vi "Log_Test.vi"() -> ()   [LabVIEW 2021]
panel:
  out "x-y":dbl
  out "Array":T1(array[cluster])
  out "string array":string[](array[string])
  out "XY Graph":T2(graph)
  in  "Stop":bool
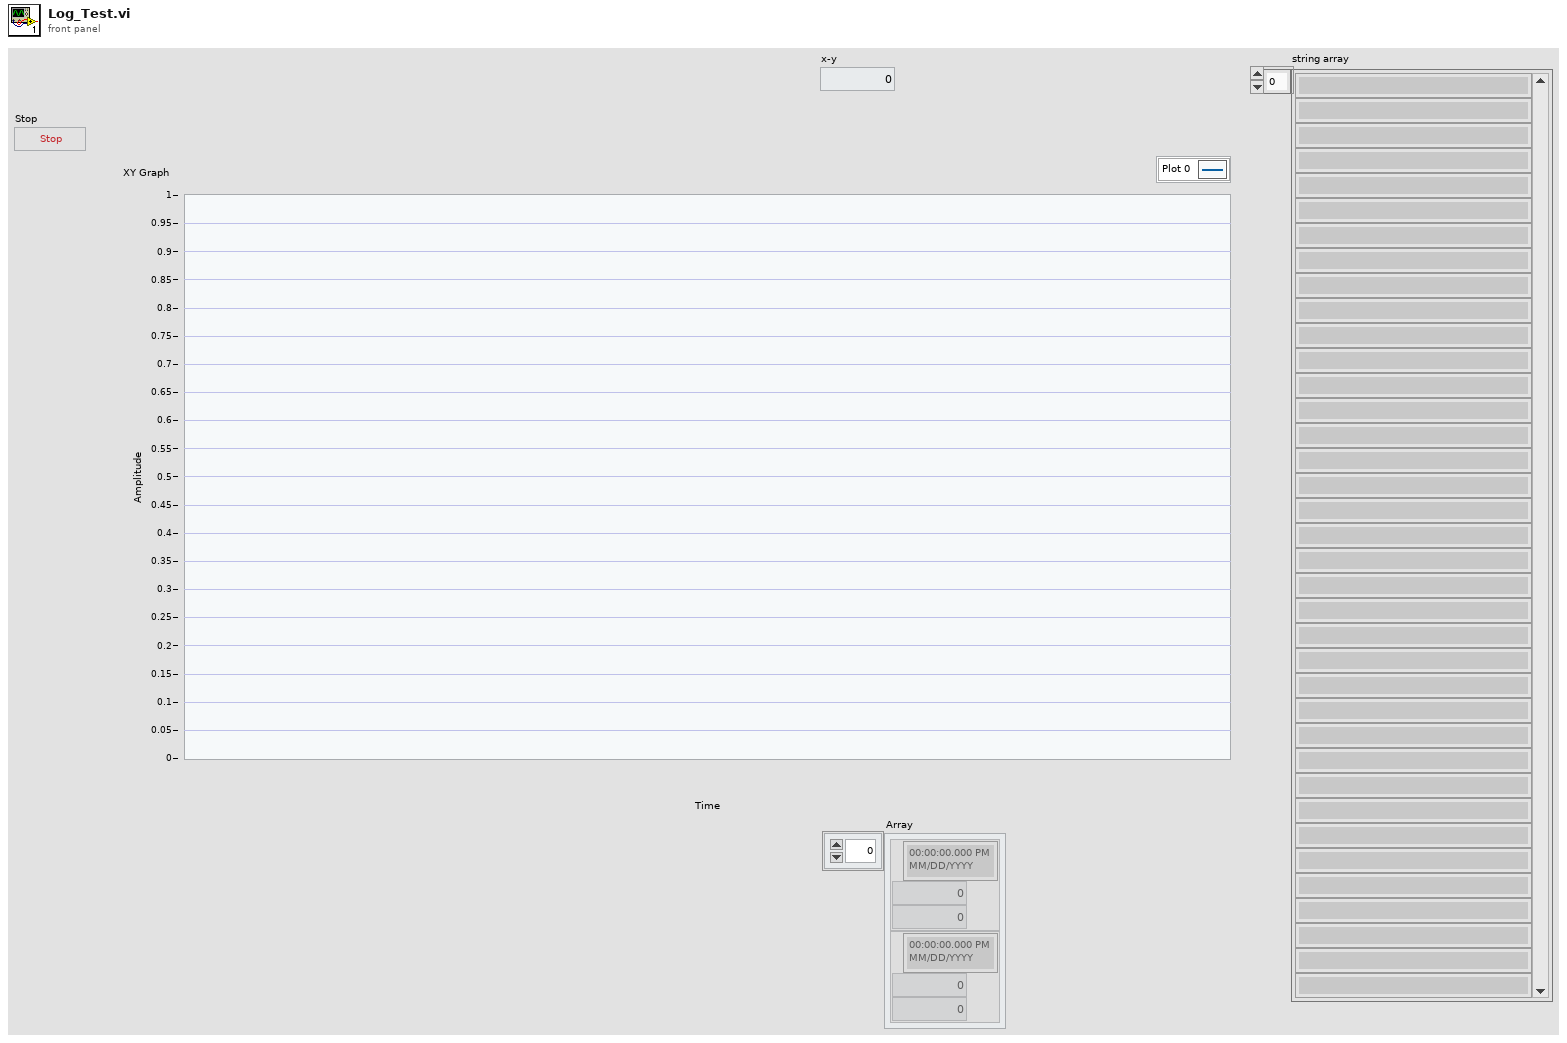
[diagram p1: front panel]
types:
  T1 = cluster{timestamp, "Numeric":dbl, "Numeric":dbl}[]
  T2 = cluster{"seconds since 1Jan1904":timestamp, "number: 0 to 1":dbl, "number: 0 to 1":dbl}[]
  T3 = enum16{"open", "replace", "create", "open or create", "replace or create", "replace or create with confirmation"}
  T4 = cluster{"seconds since 1Jan1904":timestamp, "number: 0 to 1":dbl, "number: 0 to 1":dbl}
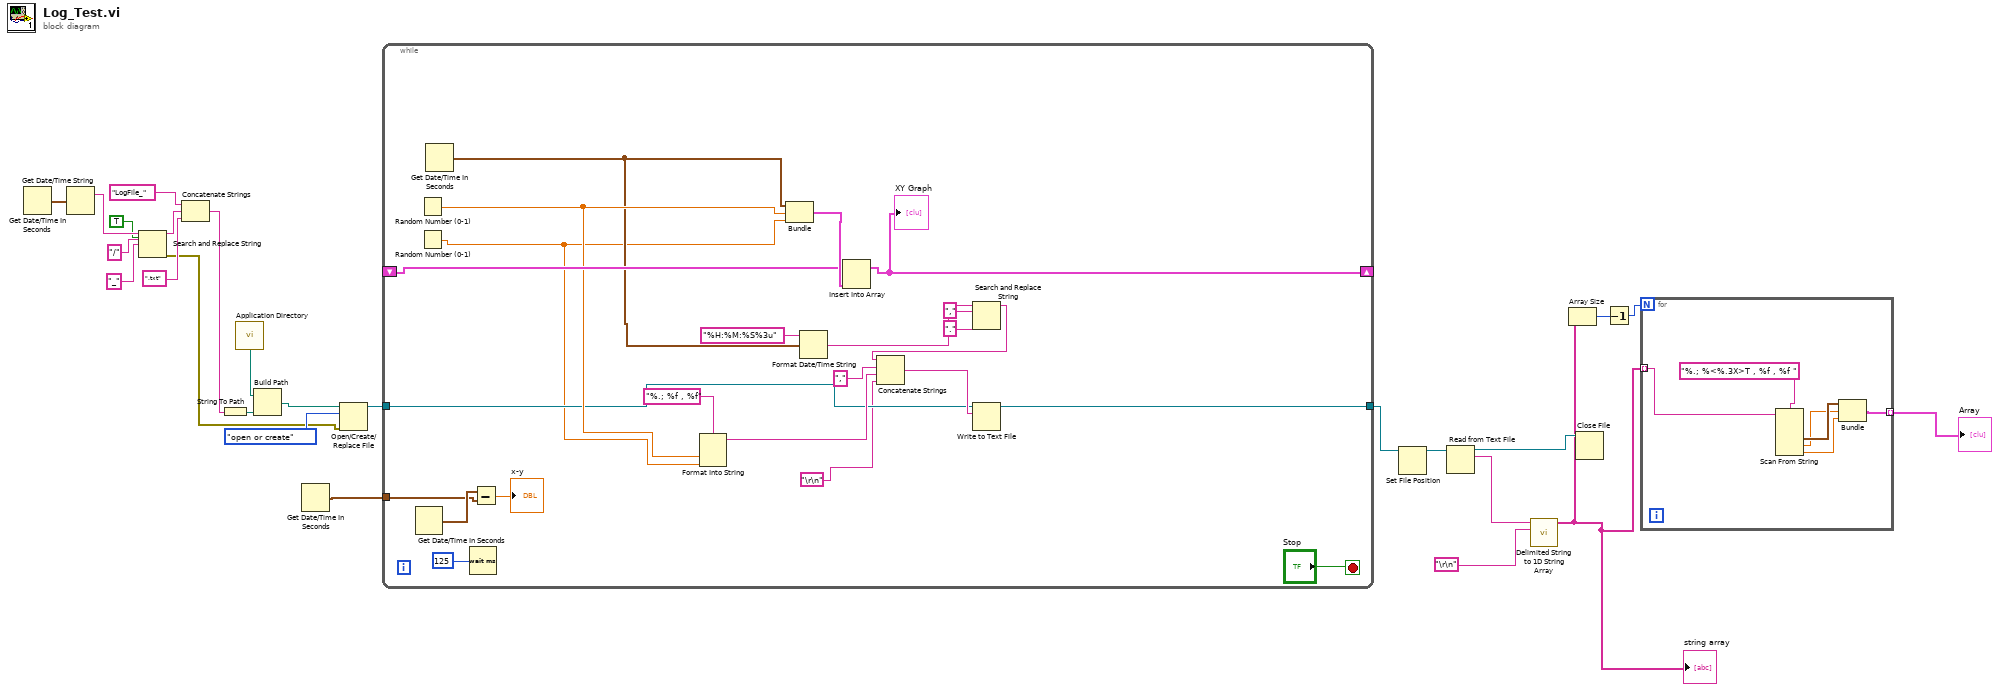
[diagram p0: block diagram]
diagram:
  n1 = Get Date/Time In Seconds() -> (seconds since 1Jan1904=w20:timestamp)
  n2 = Get Date/Time String(seconds (now)=w20) -> (date string=w19:string)  [unwired: 2 in, 1 out]
  n3 = Search and Replace String(replace all?=TRUE ("replace all? (F)"), input string=w19, search string="/", replace string="_" ("replace string (\"\")")) -> (result string=w15:string, error out=w10:errorcluster)  [unwired: 4 in, 2 out]
  n4 = Concatenate Strings("LogFile_" ("string"), w15, ".txt" ("string")) -> (w12:string)
  n5 = String To Path(string=w12) -> (path=w13:path)
  n6 = call <vilib>:"Application Directory.vi"() -> ("Application Directory"=w23:path)
  n7 = Build Path(base path=w23, name or relative path=w13) -> (appended path=w22:path)
  n8 = Get Date/Time In Seconds() -> (seconds since 1Jan1904=w1:timestamp)
  n9 = Open/Create/Replace File(file path (use dialog)=w22, error in=w10, operation (0:open)=T3."open or create") -> (refnum out=w24:refnum<file>)  [unwired: 3 in, 2 out]
  n10 = while {
    shift-right: [w45] -> _
    shift-left: _ -> [w44]
    tunnel: w24 -> [w38]
    tunnel: [w37] -> w9
    tunnel: w1 -> [w27]
    stop <- "Stop" stop-if-true
    n11 = Get Date/Time In Seconds() -> (seconds since 1Jan1904=w28:timestamp)
    n12 = Random Number (0-1)() -> (number: 0 to 1=w41:dbl)
    n13 = Random Number (0-1)() -> (number: 0 to 1=w29:dbl)
    n14 = Get Date/Time In Seconds() -> (seconds since 1Jan1904=w36:timestamp)
    n15 = Wait (ms)(milliseconds to wait=u32 125) -> ()  [unwired: 1 out]
    n16 = Subtract(x=w28, y=w27) -> (x-y=→"x-y":dbl)
    n17 = Format Into String(format string="%.; %f , %f", w41, w29) -> (resulting string=w40:string)  [unwired: 2 in, 1 out]
    n18 = Bundle("seconds since 1Jan1904"=w36, "number: 0 to 1"=w41, "number: 0 to 1"=w29) -> (w46:T4)  [unwired: 1 in]
    n19 = Format Date/Time String(time format string (%c)="%H:%M:%S%3u", seconds (now)=w36) -> (date/time string=w34:string)  [unwired: 1 in]
    n20 = Insert Into Array(array=w44, new element=w46) -> (w45:T2)  [unwired: 1 in]
    "XY Graph" <- w45
    n21 = Search and Replace String(input string=w34, search string=",", replace string="." ("replace string (\"\")")) -> (result string=w31:string)  [unwired: 5 in, 3 out]
    n22 = Concatenate Strings(w31, ",", w40, "\r\n") -> (w39:string)
    n23 = Write to Text File(file (use dialog)=w38, text=w39) -> (refnum out=w37:refnum<file>)  [unwired: 2 in, 2 out]
  }
  n24 = Set File Position(refnum=w9) -> (refnum out=w8:refnum<file>)  [unwired: 3 in, 1 out]
  n25 = Read from Text File(file (use dialog)=w8) -> (refnum out=w21:refnum<file>, text=w7:string)  [unwired: 3 in, 2 out]
  n26 = call <vilib>:"Delimited String to 1D String Array.vi"("delimiter"="\r\n", "delimited string"=w7) -> ("string array"=w4:string[])  [unwired: 9 in]
  "string array" <- w4
  n27 = Array Size(array=w4) -> (size(s)=w3:i32)
  n28 = Close File(refnum=w21) -> ()  [unwired: 1 in, 2 out]
  n29 = Decrement(x=w3) -> (x-1=w2:i32)
  n30 = for {
    N: w2 -> [_]
    tunnel: w4 -> [w53] mode=indexing
    tunnel: [w49] -> w5 mode=indexing
    n31 = Scan From String(format string="%.; %<%.3X>T , %f , %f ", input string=w53) -> (output 1=w52:timestamp, output 2=w51:dbl, output 3=w50:dbl)  [unwired: 5 in, 3 out]
    n32 = Bundle(w52, w51, w50) -> (w49:cluster{timestamp, dbl, dbl})  [unwired: 1 in]
  }
  "Array" <- w5
